vi "Create Frequency Steps Array.vi"(11 "Spectrum Recorder Configuration":T1={"Start frequency"=500000.0, "End frequency"=2000000.0, "Coarse step"=100.0, "Step duration"=0.004, "Red Pitaya address"="192.168.1.100", "Open plot \non start"=FALSE, "Fine region centers"=[], "Regions width"=2000.0, "Fine step"=1.0} {"Fine step" min=1.0 format="%#_6pHz"; "Regions width" format="%#_6pHz"; "Fine region centers" format="%#_6pHz"; "Step duration" format="%#_6ps"; "Coarse step" format="%#_6pHz"; "End frequency" format="%#_6pHz"; "Start frequency" format="%#_6pHz"}) -> (3 "Steps":dbl[](array[numeric]) format="%#_8p")   [LabVIEW 2016]
uses:
  NHMFL_Core/Libraries/Red Pitaya/RP Core/Red Pitaya Transceiver Driver/Spectrum Configuration.ctl
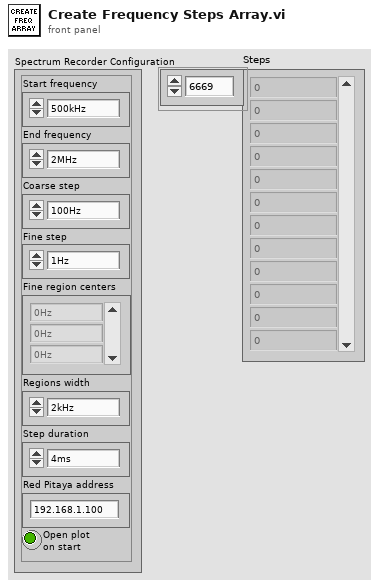
[diagram p1: front panel]
types:
  T1 = typedef "Spectrum Configuration.ctl" = cluster{"Start frequency":dbl, "End frequency":dbl, "Coarse step":dbl, "Step duration":dbl, "Red Pitaya address":string, "Open plot \non start":bool, "Fine region centers":dbl[], "Regions width":dbl, "Fine step":dbl}
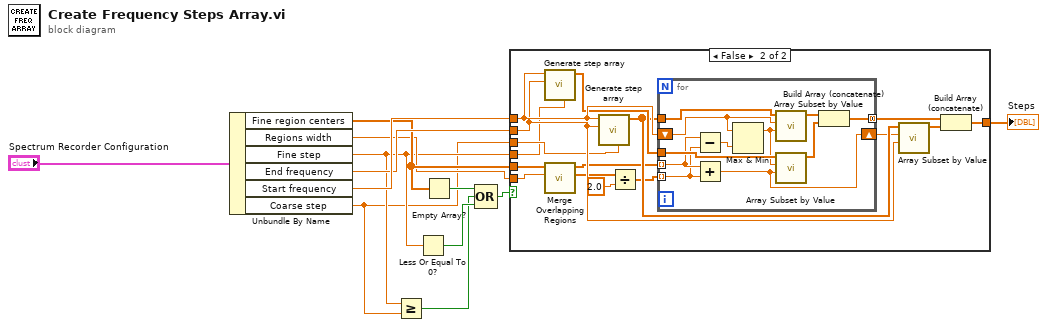
[diagram p0: block diagram]
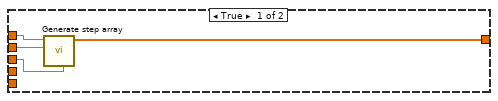
[diagram p2: hidden frame]
diagram:
  n1 = Unbundle By Name("Spectrum Recorder Configuration") -> ("Fine region centers"=w6:dbl[], "Regions width"=w5:dbl, "Fine step"=w3:dbl, "End frequency"=w11:dbl, "Start frequency"=w12:dbl, "Coarse step"=w2:dbl)
  n2 = Greater Or Equal?(x=w3, y=w2) -> (x >= y?=w1:bool)
  n3 = Less Or Equal To 0?(x=w3) -> (x <= 0?=w4:bool)
  n4 = Empty Array?(array=w6) -> (empty?=w8:bool)
  n5 = Compound Arithmetic op=OR(w8, w1, w4) -> (w7:bool)
  n6 = case shown="False" w7 {
    tunnel: [w13 w25] -> w9
    tunnel: w11 -> [w15 w28]
    tunnel: w12 -> [w16 w32]
    tunnel: w2 -> [w14 w18]
    tunnel: w3 -> [_ w17]
    tunnel: w6 -> [_ w21]
    tunnel: w5 -> [_ w24]
    frame True {
      n7 = call "Generate step array.vi"("Step"=w14, "End"=w15, "Start"=w16) -> ("Steps"=w13:dbl[])  [unwired: 8 in]
    }
    frame False {
      n8 = call "Generate step array.vi"("Step"=w17, "End"=w28, "Start"=w32) -> ("Steps"=w31:dbl[])  [unwired: 8 in]
      n9 = call "Merge Overlapping Regions.vi"("Regions width"=w24, "Region centers"=w21) -> ("Region widths out"=w22:dbl[], "Region centers out"=w20:dbl[])  [unwired: 8 in]
      n10 = call "Generate step array.vi"("Step"=w18, "End"=w28, "Start"=w32) -> ("Steps"=w30:dbl[])  [unwired: 8 in]
      n11 = Divide(x=w22, y=2.0) -> (x/y=w19:dbl[])
      n12 = for {
        tunnel: w20 -> [w41] mode=indexing
        tunnel: w30 -> [w43]
        tunnel: w19 -> [w40] mode=indexing
        shift-right: [w36] -> w29
        shift-left: w32 -> [w35]
        tunnel: w31 -> [w42]
        tunnel: [w37] -> w27 mode=concatenating
        n13 = Subtract(x=w41, y=w40) -> (x-y=w34:dbl)
        n14 = Add(x=w41, y=w40) -> (x+y=w36:dbl)
        n15 = Max & Min(x=w35, y=w34) -> (max(x,y)=w33:dbl)  [unwired: 1 out]
        n16 = call "Array Subset by Value.vi"("End"=w33, "Start"=w35, "Data"=w43) -> ("Data subset"=w39:dbl[])  [unwired: 8 in]
        n17 = call "Array Subset by Value.vi"("End"=w36, "Start"=w33, "Data"=w42) -> ("Data subset"=w38:dbl[])  [unwired: 8 in]
        n18 = Build Array (concatenate)(w39, w38) -> (w37:dbl[])
      }
      n19 = call "Array Subset by Value.vi"("End"=w28, "Start"=w29, "Data"=w30) -> ("Data subset"=w26:dbl[])  [unwired: 8 in]
      n20 = Build Array (concatenate)(w27, w26) -> (w25:dbl[])
    }
  }
  "Steps" <- w9
